vi "Filter Data Clear.vi"(8 "error in (no error)":errorcluster, 11 "Post Analysis in":refnum<class "Post Analysis.lvclass">) -> (0 "error out":errorcluster, 3 "Post Analysis out":refnum<class "Post Analysis.lvclass">)   [LabVIEW 2023, in "Data Analysis.lvlib" / "Post Analysis.lvlib" / "Post Analysis.lvclass"]
uses:
  Post Analysis.lvclass
  Post Analysis.lvclass/Post Analysis.ctl
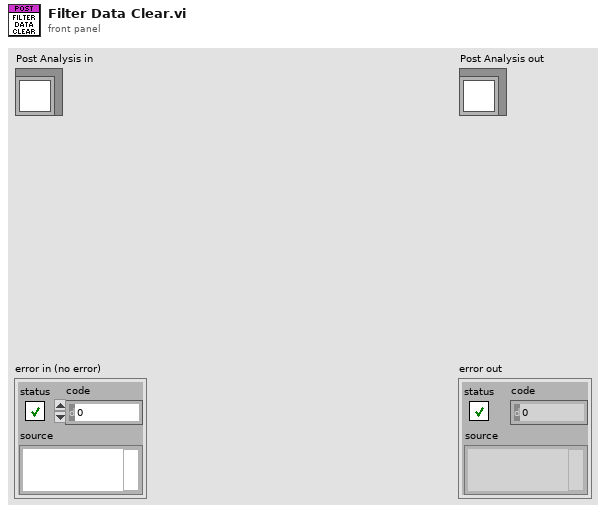
[diagram p1: front panel]
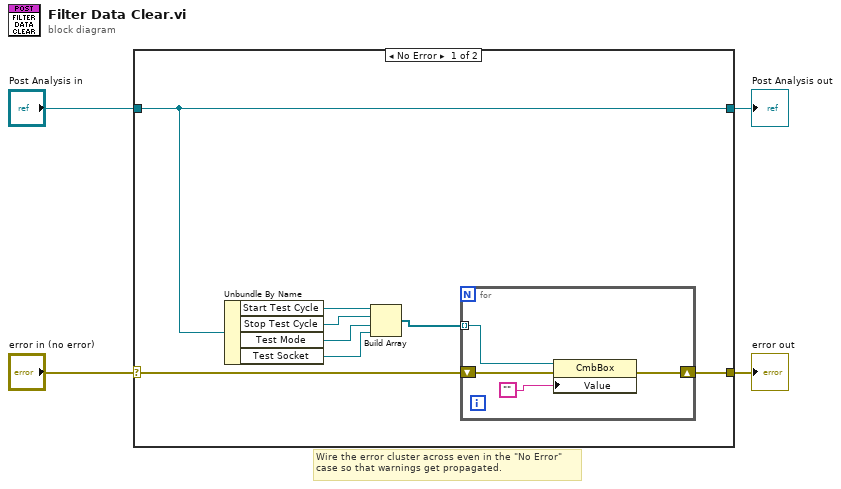
[diagram p0: block diagram]
diagram:
  # "Wire the error cluster across even in the \"No Error\"\ncase so that warnings get propagated."
  n1 = case shown="No Error" "error in (no error)" {
    selector: "error in (no error)" -> [w6 w18]
    tunnel: [w5 w18] -> w3
    tunnel: [w12 w17] -> w1
    tunnel: "Post Analysis in" -> [w12 w17]
    frame No Error {
      n2 = Unbundle By Name(w12) -> ("Start Test Cycle"=w11:refnum<vi>, "Stop Test Cycle"=w10:refnum<vi>, "Test Mode"=w9:refnum<vi>, "Test Socket"=w8:refnum<vi>)
      n3 = Build Array(w11, w10, w9, w8) -> (w7:refnum<vi>[])
      n4 = for {
        tunnel: w7 -> [w16] mode=indexing
        shift-right: [w13] -> w5
        shift-left: w6 -> [w14]
        n5 = property class="CmbBox"(reference=w16, error in=w14, "Value"="") -> (error out=w13:errorcluster)  [unwired: 1 out]
      }
    }
    frame Error {
    }
  }
  "error out" <- w3
  "Post Analysis out" <- w1
